vi "Configure Modulation (Phase).vi"(0 "VISA resource name":refnum<visa-resource-name>, 1 "Phase Modulation Frequency (100.00  Hz)":dbl=100.0 min=0.002 max=20000.0 format="%.2f", 2 "Phase Deviation (180 deg)":dbl=180.0 min=0.0 max=360.0 format="%.1f", 5 "Enable Phase Modulation  (T: Enable)":bool=TRUE, 7 "Phase Modulation Source (0: Internal)":u16(ring) items=["Internal", "External"], 9 "Modulation Waveform (0: Sine)":i32(ring) items=["Sine", "Square", "Ramp", "Negative Ramp", "Triangle", "Noise", "Arbitrary Waveform"], 11 "error in (no error)":errorcluster) -> (4 "VISA resource name out":refnum<visa-resource-name>, 15 "error out":errorcluster)   [LabVIEW 2012, in "Agilent 33XXX Series.lvlib"]
doc: "Allows and configures phase modulation. The phase of the carrier is varied by the amplitude of the modulating waveform. The carrier waveform shape and parameters are set by config waveform function.\n\nNote:\n(1) This VI is only used with the Agilent 33210A and 33220A.\n(2) Before using this mode, all other modes must be turned off.\n(3) The carrier waveform shape and parameters are set by the Configure Standard Waveform VI."
uses:
  <instrlib>/Agilent 33XXX Series/Agilent 33XXX Series.lvlib
panel:
  # "Internal Phase Modulation Settings"
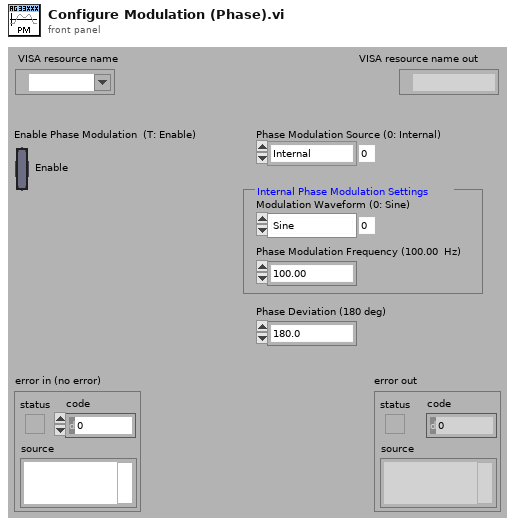
[diagram p1: front panel]
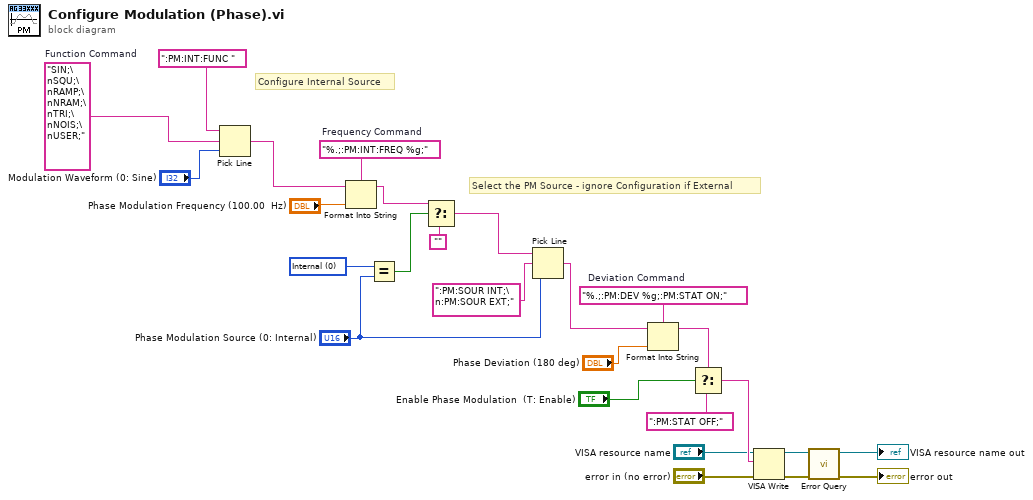
[diagram p0: block diagram]
diagram:
  w17 = "SIN;\nSQU;\nRAMP;\nNRAM;\nTRI;\nNOIS;\nUSER;"  # Function Command
  w19 = "%.;:PM:INT:FREQ %g;"  # Frequency Command
  w23 = "%.;:PM:DEV %g;:PM:STAT ON;"  # Deviation Command
  w8 = u16 0 items=["Internal", "External"] ("Source (0: Internal)")
  # "Configure Internal Source"
  # "Select the PM Source - ignore Configuration if External"
  n1 = Pick Line(string ("")=":PM:INT:FUNC ", multi-line string=w17, line index="Modulation Waveform (0: Sine)") -> (output string=w18:string)
  n2 = Format Into String(format string=w19, initial string=w18, "Phase Modulation Frequency (100.00  Hz)") -> (resulting string=w12:string)  [unwired: 1 in, 1 out]
  n3 = Equal?(x=w8, y="Phase Modulation Source (0: Internal)") -> (x = y?=w13:bool)
  n4 = Select(t=w12, s=w13, f="") -> (s? t:f=w10:string)
  n5 = Pick Line(string ("")=w10, multi-line string=":PM:SOUR INT;\n:PM:SOUR EXT;" ("Source Command"), line index="Phase Modulation Source (0: Internal)") -> (output string=w9:string)
  n6 = Format Into String(format string=w23, initial string=w9, "Phase Deviation (180 deg)") -> (resulting string=w15:string)  [unwired: 1 in, 1 out]
  n7 = Select(t=w15, s="Enable Phase Modulation  (T: Enable)", f=":PM:STAT OFF;") -> (s? t:f=w6:string)
  n8 = VISA Write(VISA resource name="VISA resource name", write buffer=w6, error in (no error)="error in (no error)") -> (VISA resource name out=w26:refnum<visa-resource-name>, error out=w25:errorcluster)  [unwired: 1 out]
  n9 = call <instrlib>:"Error Query.vi"("error in (no error)"=w25, "VISA resource name"=w26) -> ("error out"=→"error out":errorcluster, "VISA resource name out"=→"VISA resource name out":refnum<visa-resource-name>)  [unwired: 6 in, 2 out]
